vi "CheckIfConnectorPanesMatch.vi"(8 "error in (no error)":errorcluster, 10 "actual connector pane vi":path, 11 "expected connector pane vi":path) -> (0 "error out":errorcluster, 1 "mismatch explanation":string, 3 "connector panes match":bool)   [LabVIEW 2015, in "VeriStandTestCase.lvclass"]
uses:
  VeriStandTestCase.lvclass
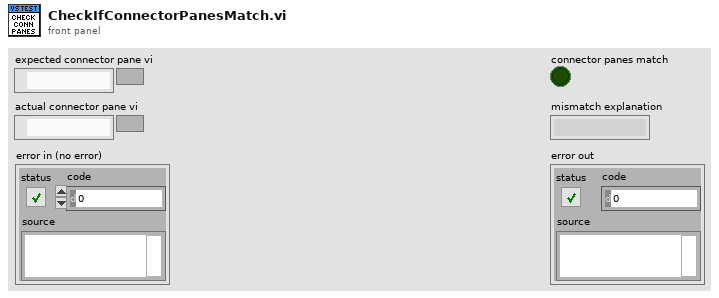
[diagram p1: front panel]
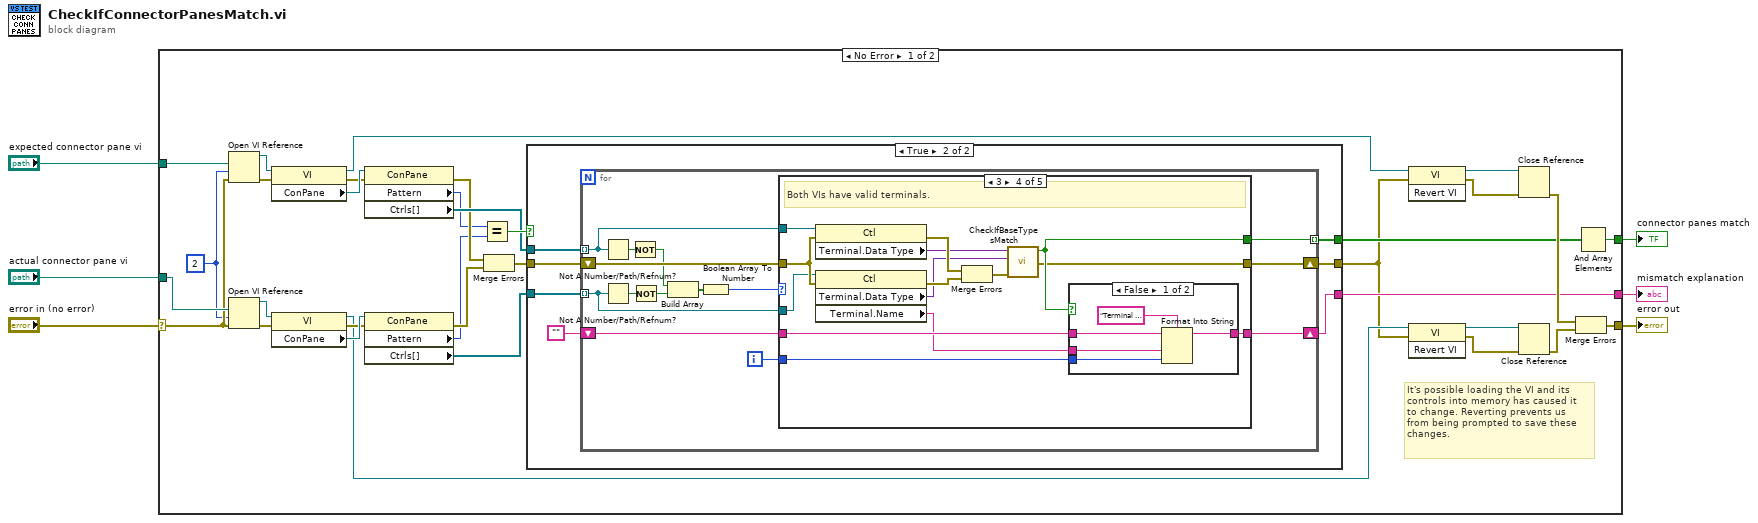
[diagram p0: block diagram]
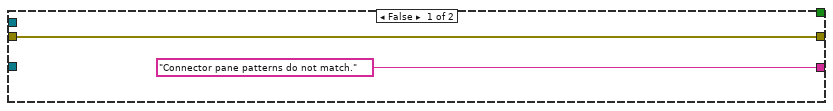
[diagram p2: hidden frame]
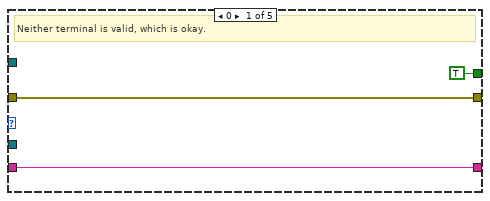
[diagram p3: hidden frame]
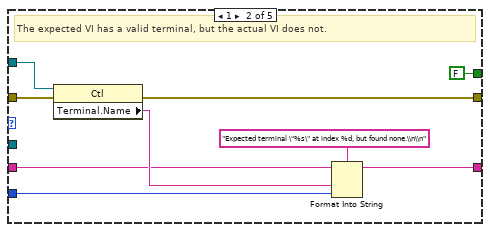
[diagram p4: hidden frame]
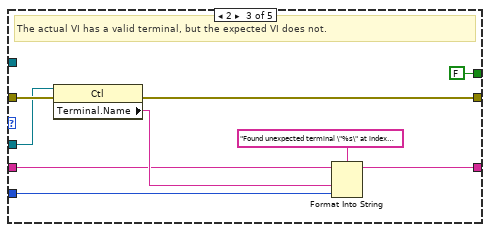
[diagram p5: hidden frame]
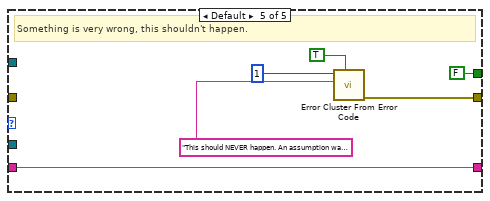
[diagram p7: hidden frame]
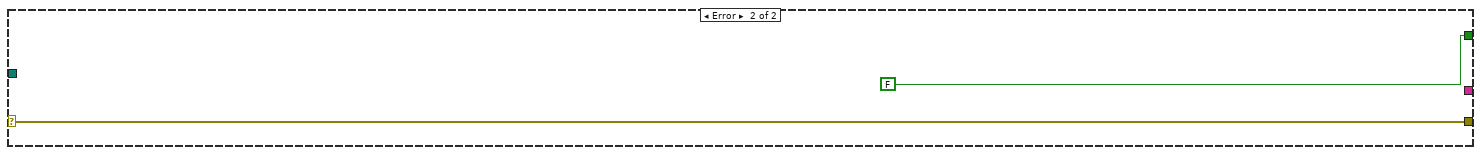
[diagram p8: hidden frame]
diagram:
  n1 = case shown="No Error" "error in (no error)" {
    selector: "error in (no error)" -> [w31 w111]
    tunnel: "actual connector pane vi" -> [w39 _]
    tunnel: "expected connector pane vi" -> [w33 _]
    tunnel: [w20 w111] -> w3
    tunnel: [w19 FALSE] -> w2
    tunnel: [w15 _] -> w1
    frame No Error {
      w14 = 2 ("options")
      # "It's possible loading the VI and its\ncontrols into memory has caused it\nto change. Reverting prevents us\nfrom being prompted to save these\nchanges."
      n2 = Open VI Reference(vi path=w33, options=w14, error in (no error)=w31) -> (vi reference=w34:refnum<vi>, error out=w35:errorcluster)  [unwired: 3 in]
      n3 = Open VI Reference(vi path=w39, options=w14, error in (no error)=w31) -> (vi reference=w38:refnum<vi>, error out=w37:errorcluster)  [unwired: 3 in]
      n4 = property class="VI"(reference=w34, error in=w35) -> (reference out=w7:refnum<vi>, error out=w26:errorcluster, "ConPane"=w32:refnum<vi>)
      n5 = property class="VI"(reference=w38, error in=w37) -> (reference out=w12:refnum<vi>, error out=w27:errorcluster, "ConPane"=w36:refnum<vi>)
      n6 = property class="ConPane"(reference=w32, error in=w26) -> (error out=w25:errorcluster, "Pattern"=w17:u32, "Ctrls[]"=w29:refnum<vi>[])  [unwired: 1 out]
      n7 = property class="ConPane"(reference=w36, error in=w27) -> (error out=w24:errorcluster, "Pattern"=w18:u32, "Ctrls[]"=w28:refnum<vi>[])  [unwired: 1 out]
      n8 = Equal?(x=w17, y=w18) -> (x = y?=w30:bool)
      n9 = Merge Errors(w25, w24) -> (w23:errorcluster)
      n10 = case shown="True" w30 {
        tunnel: w28 -> [_ w48]
        tunnel: w29 -> [_ w47]
        tunnel: w23 -> [w41 w46]
        tunnel: [w41 w45] -> w9
        tunnel: [_ w44] -> w16
        tunnel: ["Connector pane patterns do not match." w42] -> w15
        frame False {
        }
        frame True {
          n11 = for {
            tunnel: w48 -> [w50] mode=indexing
            tunnel: w47 -> [w51] mode=indexing
            tunnel: [w52] -> w44 mode=indexing
            shift-right: [w57] -> w45
            shift-left: w46 -> [w58]
            shift-right: [w55] -> w42
            shift-left: "" -> [w56]
            i -> [w49]
            n12 = Not A Number/Path/Refnum?(number/path/refnum=w51) -> (NaN/Path/Refnum?=w62:bool)
            n13 = Not A Number/Path/Refnum?(number/path/refnum=w50) -> (NaN/Path/Refnum?=w61:bool)
            n14 = Not(x=w62) -> (.not. x?=w54:bool)
            n15 = Not(x=w61) -> (.not. x?=w53:bool)
            n16 = Build Array(w54, w53) -> (w60:bool[])
            n17 = Boolean Array To Number(Boolean array=w60) -> (number=w59:u32)
            n18 = case shown="3" w59 {
              tunnel: w58 -> [w65 w72 w80 w94 _]
              tunnel: [w65 w71 w81 w84 w109] -> w57
              tunnel: w56 -> [w64 w70 w77 w93 w107]
              tunnel: [w64 w69 w76 w92 w107] -> w55
              tunnel: [TRUE FALSE FALSE w86 FALSE] -> w52
              tunnel: w51 -> [_ w73 _ w90 _]
              tunnel: w50 -> [_ _ w79 w89 _]
              tunnel: w49 -> [_ w67 w78 w91 _]
              frame 0 {
                # "Neither terminal is valid, which is okay."
              }
              frame 1 {
                # "The expected VI has a valid terminal, but the actual VI does not."
                n19 = property class="Ctl"(reference=w73, error in=w72) -> (error out=w71:errorcluster, "Terminal.Name"=w74:string)  [unwired: 1 out]
                n20 = Format Into String(format string="Expected terminal \"%s\" at index %d, but found none.\\n\\n", initial string=w70, w74, w67) -> (resulting string=w69:string)  [unwired: 1 in, 1 out]
              }
              frame 2 {
                # "The actual VI has a valid terminal, but the expected VI does not."
                n21 = property class="Ctl"(reference=w79, error in=w80) -> (error out=w81:errorcluster, "Terminal.Name"=w83:string)  [unwired: 1 out]
                n22 = Format Into String(format string="Found unexpected terminal \"%s\" at index %d, expected none.\\n\\n", initial string=w77, w83, w78) -> (resulting string=w76:string)  [unwired: 1 in, 1 out]
              }
              frame 3 {
                # "Both VIs have valid terminals."
                n23 = property class="Ctl"(reference=w90, error in=w94) -> (error out=w97:errorcluster, "Terminal.Data Type"=w95:variant)  [unwired: 1 out]
                n24 = property class="Ctl"(reference=w89, error in=w94) -> (error out=w96:errorcluster, "Terminal.Data Type"=w87:variant, "Terminal.Name"=w88:string)  [unwired: 1 out]
                n25 = Merge Errors(w97, w96) -> (w85:errorcluster)
                n26 = call "CheckIfBaseTypesMatch.vi"("error in (no error)"=w85, "Actual data type"=w87, "Expected data type"=w95) -> ("error out"=w84:errorcluster, "types match"=w86:bool)  [unwired: 7 in]
                n27 = case shown="False" w86 {
                  tunnel: [w102 w103] -> w92
                  tunnel: w93 -> [w99 w103]
                  tunnel: w91 -> [w100 _]
                  tunnel: w88 -> [w98 _]
                  frame False {
                    n28 = Format Into String(format string="Terminal \"%s\" at index %d does not have expected type.\\n\\n", initial string=w99, w98, w100) -> (resulting string=w102:string)  [unwired: 1 in, 1 out]
                  }
                  frame True {
                  }
                }
              }
              frame Default {
                # "Something is very wrong, this shouldn't happen."
                n29 = call <vilib>:"Error Cluster From Error Code.vi"("show call chain? (False)"=TRUE, "error message (\"\")"="This should NEVER happen. An assumption was made that exactly two boolean statements were being checked together; either this has been changed, or a case has been removed and not handled properly." ("error message (\"\")"), "error code (0)"=1) -> ("error out"=w109:errorcluster)  [unwired: 6 in]
              }
            }
          }
        }
      }
      n30 = invoke class="VI" method="Revert VI"(reference=w7, error in=w9) -> (reference out=w8:refnum<vi>, error out=w10:errorcluster)  [unwired: 1 in, 1 out]
      n31 = invoke class="VI" method="Revert VI"(reference=w12, error in=w9) -> (reference out=w13:refnum<vi>, error out=w11:errorcluster)  [unwired: 1 in, 1 out]
      n32 = Close Reference(reference=w8, error in (no error)=w10) -> (error out=w21:errorcluster)
      n33 = Close Reference(reference=w13, error in (no error)=w11) -> (error out=w22:errorcluster)
      n34 = Merge Errors(w21, w22) -> (w20:errorcluster)
      n35 = And Array Elements(Boolean array=w16) -> (logical AND=w19:bool)
    }
    frame Error {
    }
  }
  "error out" <- w3
  "connector panes match" <- w2
  "mismatch explanation" <- w1
